vi "Lancing Math Algo.vi"(0 "Wm":dbl format="%#_13g", 1 "Curl Gap":dbl format="%#_13g", 5 "Hm":dbl format="%#_13g", 7 "sin_net":dbl format="%#_13g", 9 "cos_net":dbl format="%#_13g", 11 "Hm'":dbl, 12 "Lock Width":dbl=2.1 format="%#_13g") -> (4 "Lancing":dbl)   [LabVIEW 2019, in "Algorithm.lvclass"]
uses:
  FrameworkOverrides/Algorithm.lvclass
panel:
  out "H":dbl
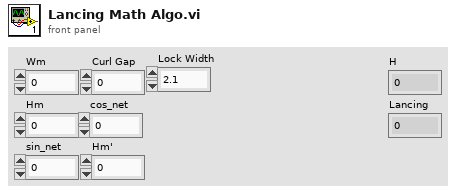
[diagram p1: front panel]
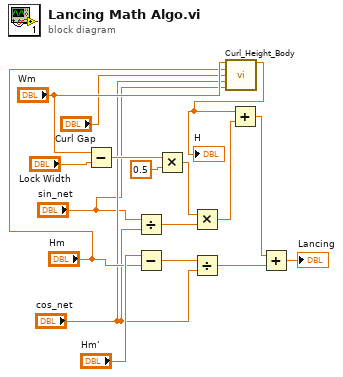
[diagram p0: block diagram]
diagram:
  n1 = Subtract(x="Wm", y="Lock Width") -> (x-y=w11:dbl)
  n2 = Divide(x="sin_net", y="cos_net") -> (x/y=w16:dbl)
  n3 = Subtract(x="Hm'", y="Hm") -> (x-y=w8:dbl)
  n4 = Multiply(x=w11, y=0.5) -> (x*y=w9:dbl)
  n5 = Multiply(x=w9, y=w16) -> (x*y=w15:dbl)
  n6 = Divide(x=w8, y="cos_net") -> (x/y=w7:dbl)
  n7 = call "Curl_Height_Body.vi"("Wm"="Wm", "Hm"="Hm", "Curl Gap"="Curl Gap", "cos_net"="cos_net", "sin_net"="sin_net") -> ("H"=w1:dbl)  [unwired: 10 in]
  "H" <- w1
  n8 = Add(x=w1, y=w15) -> (x+y=w14:dbl)
  n9 = Add(x=w14, y=w7) -> (x+y=→"Lancing":dbl)
